vi "LS372_Open_Queue.vi"() -> (2 "queue out":refnum<queue>)   [LabVIEW 2016]
uses:
  Gustav/20TVTI_Control.ctl
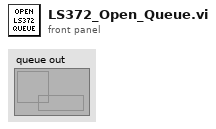
[diagram p1: front panel]
types:
  T1 = typedef "20TVTI_Control.ctl" = cluster{"Set VTI SP":bool, "Change NV Status":bool, "Set NV Setpoint":bool, "Change Heater Status":bool, "Set D-Heater Setpoint":bool, "Set Heater Setpoint":bool, "Change D-Heater Status":bool, "Set Sweep Type":bool, "Setpoint (K)":dbl, "Rate (K/min)":dbl, "Setpoint Heater":dbl, "Setpoint D-Heater":dbl, "Setpoint NV":dbl}
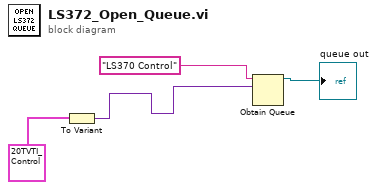
[diagram p0: block diagram]
diagram:
  n1 = To Variant(anything=T1 {"Set VTI SP"=FALSE, "Change NV Status"=FALSE, "Set NV Setpoint"=FALSE, "Change Heater Status"=FALSE, "Set D-Heater Setpoint"=FALSE, "Set Heater Setpoint"=FALSE, "Change D-Heater Status"=FALSE, "Set Sweep Type"=FALSE, "Setpoint (K)"=0.0, "Rate (K/min)"=0.0, "Setpoint Heater"=0.0, "Setpoint D-Heater"=0.0, "Setpoint NV"=0.0} ("Cluster")) -> (Variant=w3:variant)
  n2 = Obtain Queue(name (unnamed)="LS370 Control", element data type=w3) -> (queue out=→"queue out":refnum<queue>)  [unwired: 3 in, 2 out]
